vi "libtiff 32 64.vi"() -> ()   [LabVIEW 2012]
doc: "SciScan 1.2 160622"
panel:
  in  "32 or 64bit? (T:32 F:64)":bool
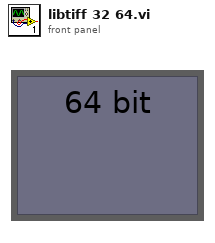
[diagram p1: front panel]
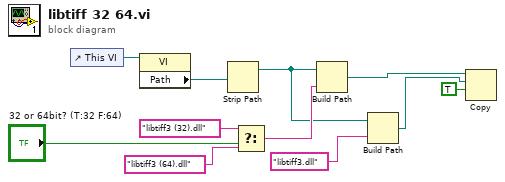
[diagram p0: block diagram]
diagram:
  n1 = control-ref of="This VI"() -> (w11:refnum<vi>)
  n2 = property class="VI"(reference=w11) -> ("Path"=w10:path)  [unwired: 1 in, 2 out]
  n3 = Strip Path(path=w10) -> (stripped path=w3:path)  [unwired: 1 out]
  n4 = Select(t="libtiff3 (32).dll", s="32 or 64bit? (T:32 F:64)", f="libtiff3 (64).dll" ("name or relative path")) -> (s? t:f=w6:string)
  n5 = Build Path(base path=w3, name or relative path=w6) -> (appended path=w4:path)
  n6 = Build Path(base path=w3, name or relative path="libtiff3.dll") -> (appended path=w1:path)
  n7 = Copy(9:TRUE ("overwrite (F)"), 10:w1, 11:w4) -> ()  [unwired: 2 in, 3 out]
